vi "Codec_CMD_23.vi"(8 "error in (no error)":errorcluster, 10 "AskCMD23":T1={"STATION"="F/T-B", "RACK"="101", "DUT"="1", "SN"="AP32023099", "DESC"="Testing PASS", "RESULT"="PASS", "SET_RACK_STATUS"="OPEN"}, 11 "SecureMqttCodec in":refnum<class "SecureMqttCodec.lvclass">) -> (0 "error out":errorcluster, 2 "<JSON>":string="{\r  \"CMD\": 23,\r  \"CONTENT\": [\r    {\r      \"DESC\": \"Testing PASS\",\r      \"DUT\": \"1\",\r      \"RACK\": \"101\",\r      \"REQ_ID\": \"BBD86106-8C6F-4C11-ABB7-FE0D978094D7\",\r      \"RESULT\": \"PASS\",\r      \"SET_RACK_STATUS\": \"OPEN\",\r      \"SN\": \"AP32023099\",\r      \"STATION\": \"F/T-B\"\r    }\r  ],\r  \"ERRCODE\": \"\",\r  \"ERRMSG\": \"\",\r  \"FROM\": \"845CF3525B43\",\r  \"ID\": \"BBD86106-8C6F-4C11-ABB7-FE0D978094D7\",\r  \"STATUS\": \"\",\r  \"TIMESTAMP\": 1759591935,\r  \"TO\": \"\"\r}", 3 "SecureMqttCodec out":refnum<class "SecureMqttCodec.lvclass">)   [LabVIEW 2020, in "SecureMqttCodec.lvclass"]
uses:
  SecureMqttCodec.lvclass
  <vilib>/addons/JSON API/JSON Object/JSON Object.lvclass
  <vilib>/addons/JSON API/JSON Scalar/JSON Scalar.lvclass
  C:/Program Files/National Instruments/LabVIEW 2020/vi.lib/addons/JSON API/JSON Value/JSON Value.lvclass
  TestMQTT/Ctrl/ReplyCMD23.ctl
  SecureMqttCodec.lvclass/SecureMqttCodec.ctl
  <vilib>/addons/JSON API/JSON Value/Set from JSON string.vi
  <vilib>/addons/JSON API/JSON Array/JSON Array.lvclass
  <vilib>/addons/JSON API/JSON Value/Set Item by name array.vi
  <vilib>/addons/JSON API/JSON Value/JSON Value.lvclass
  <vilib>/addons/JSON API/JSON Scalar/Set U32.vi
  <vilib>/addons/JSON API/JSON Value/Get Object Item by Name.vi
  <vilib>/addons/JSON API/JSON Value/Set sub-Item by names.vi
  <vilib>/addons/JSON API/JSON Array/Set JSON Array.vi
  <vilib>/addons/JSON API/JSON Value/Get as JSON string (pretty).vi
  <vilib>/addons/JSON API/Get Polymorphic/JSON GetSet.lvlib
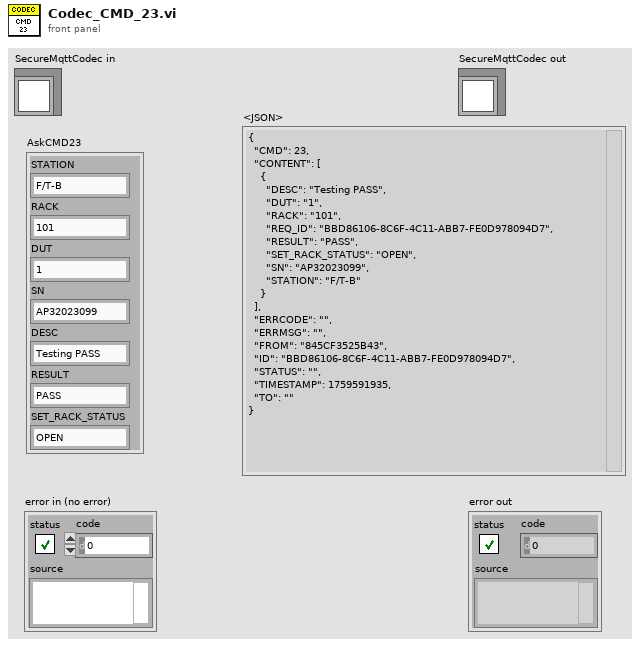
[diagram p1: front panel]
types:
  T1 = typedef "ReplyCMD23.ctl" = cluster{"STATION":string, "RACK":string, "DUT":string, "SN":string, "DESC":string, "RESULT":string, "SET_RACK_STATUS":string}
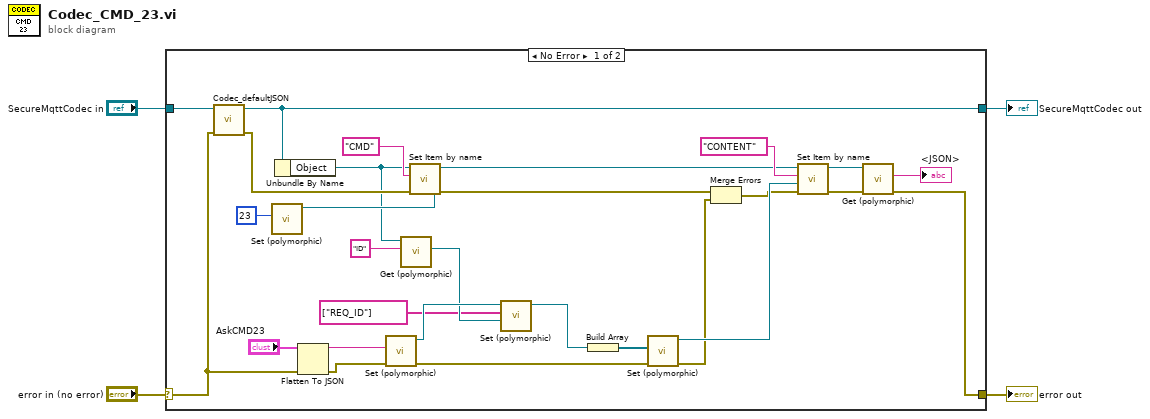
[diagram p0: block diagram]
diagram:
  n1 = case shown="No Error" "error in (no error)" {
    selector: "error in (no error)" -> [w16 w34]
    tunnel: [w29 w34] -> w3
    tunnel: [w22 w33] -> w1
    tunnel: "SecureMqttCodec in" -> [w32 w33]
    frame No Error {
      n2 = call "Codec_defaultJSON.vi"("error in (no error)"=w16, "SecureMqttCodec in"=w32) -> ("error out"=w21:errorcluster, "SecureMqttCodec out"=w22:refnum<class "SecureMqttCodec.lvclass">)  [unwired: 8 in]
      n3 = call-poly <vilib>:"Set (polymorphic).vi"("Numeric"=u32 23) -> ("JSON Scalar out"=w30:refnum<class "JSON Scalar.lvclass">)  [unwired: 9 in, 1 out]
      n4 = Unbundle By Name(w22) -> ("Object"=w10:refnum<class "JSON Value.lvclass">)
      n5 = Flatten To JSON(anything="AskCMD23", error in (no error)=w16) -> (JSON string=w18:string, 11:w17:errorcluster)  [unwired: 1 in]
      n6 = call-poly <vilib>:"Set (polymorphic).vi"("error in (no error)"=w17, "JSON stream"=w18) -> ("error out"=w15:errorcluster, "JSON Value out"=w8:refnum<class "JSON Value.lvclass">)  [unwired: 7 in, 1 out]
      n7 = call-poly <vilib>:"Get (polymorphic).vi"("name"="ID" ("String"), "JSON Value In"=w10) -> ("Value"=w7:refnum<class "JSON Value.lvclass">)  [unwired: 6 in, 3 out]
      n8 = call-dynamic "Set Item by name.vi"("error in (no error)"=w21, "Value"=w30, "name"="CMD", "JSON Value In"=w10) -> ("error out"=w26:errorcluster, "JSON Value Out"=w11:refnum<class "JSON Value.lvclass">)  [unwired: 5 in, 1 out]
      n9 = call-poly <vilib>:"Set (polymorphic).vi"("Value"=w7, "Name Array"=string[] ["REQ_ID"], "JSON Value In"=w8) -> ("JSON Value Out"=w5:refnum<class "JSON Value.lvclass">)  [unwired: 6 in, 2 out]
      n10 = Build Array(w5) -> (w19:refnum<class "JSON Value.lvclass">[])
      n11 = call-poly <vilib>:"Set (polymorphic).vi"("error in (no error)"=w15, "Array"=w19) -> ("error out"=w13:errorcluster, "JSON Array out"=w24:refnum<class "JSON Array.lvclass">)  [unwired: 8 in]
      n12 = Merge Errors(w26, w13) -> (w14:errorcluster)
      n13 = call-dynamic "Set Item by name.vi"("error in (no error)"=w14, "Value"=w24, "name"="CONTENT", "JSON Value In"=w11) -> ("error out"=w25:errorcluster, "JSON Value Out"=w27:refnum<class "JSON Value.lvclass">)  [unwired: 5 in, 1 out]
      n14 = call-poly <vilib>:"Get (polymorphic).vi"("error in (no error)"=w25, "JSON Value in"=w27) -> ("error out"=w29:errorcluster, "<JSON>"=→"<JSON>":string)  [unwired: 8 in]
    }
    frame Error {
    }
  }
  "error out" <- w3
  "SecureMqttCodec out" <- w1
